vi "CreatePostUUTSequence.vi"(0 "Engine In":refnum<k7>, 5 "NewSequenceFile in":refnum<k7>, 11 "Error In":errorcluster) -> (4 "Engine Out":refnum<k7>, 6 "NewSequenceFile out":refnum<k7>, 15 "Error Out":errorcluster)   [LabVIEW 2021, in "Create Sequence.lvlib"]
uses:
  Create Sequence.lvlib
  TypeDef/StepProperties.ctl
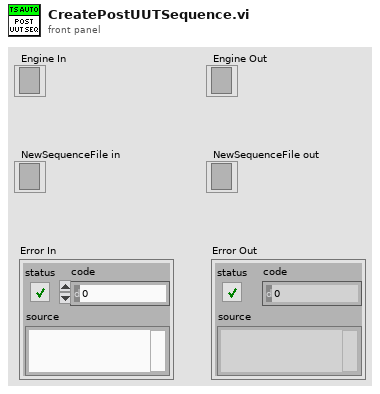
[diagram p1: front panel]
types:
  T1 = typedef "Create Sequence.lvlib/StepProperties.ctl" = cluster{"StepTypeName":string, "StepName":string, "Description":string, "Comment":string, "sequenceNameParam":string, "Step Group":i32, "Step Index":i32, "Expression":string}
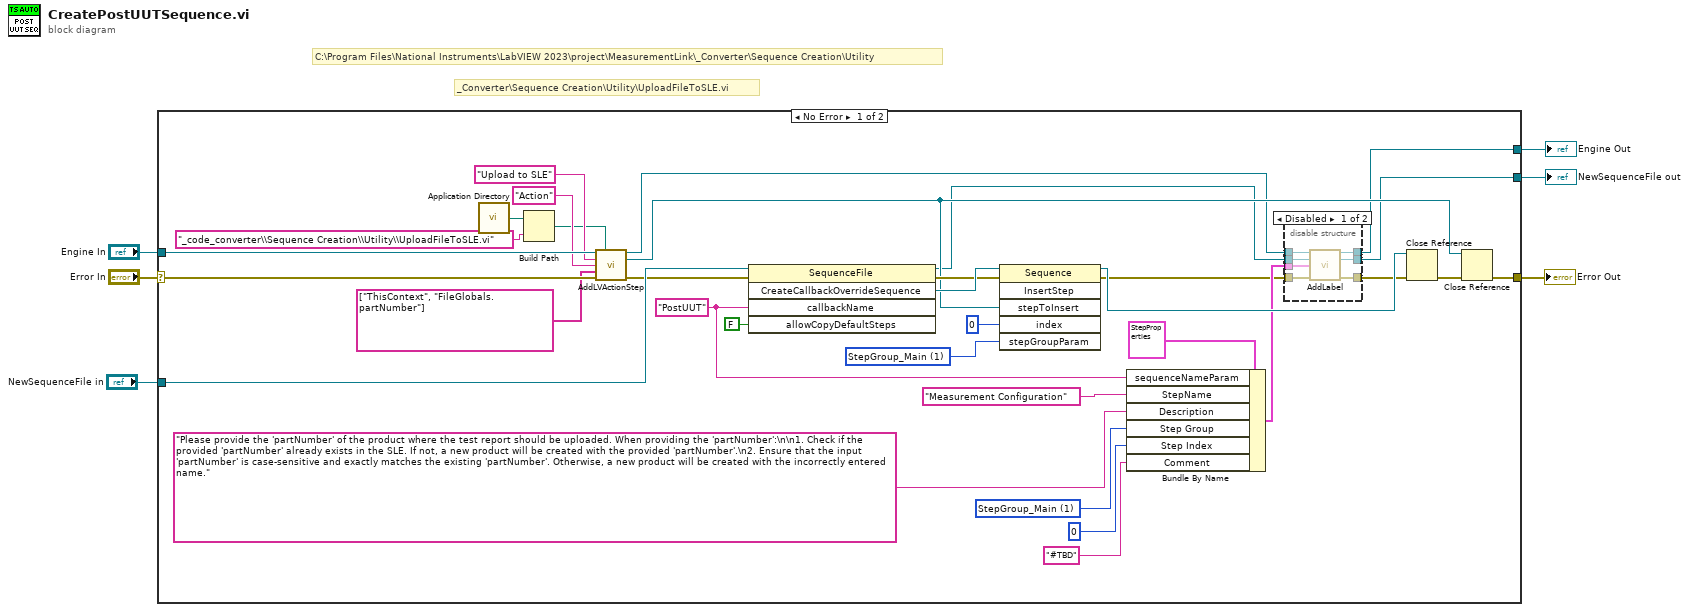
[diagram p0: block diagram]
diagram:
  # "_Converter\\Sequence Creation\\Utility\\UploadFileToSLE.vi"
  # "C:\\Program Files\\National Instruments\\LabVIEW 2023\\project\\MeasurementLink\\_Converter\\Sequence Creation\\Utility"
  n1 = case shown="No Error" "Error In" {
    selector: "Error In" -> [w35 w52]
    tunnel: [w37 w52] -> w6
    tunnel: [w11 w50] -> w5
    tunnel: [w13 w51] -> w4
    tunnel: "NewSequenceFile in" -> [w25 w50]
    tunnel: "Engine In" -> [w36 w51]
    frame No Error {
      w19 = 1 items=["StepGroup_Setup", "StepGroup_Main", "StepGroup_Cleanup"] ("Step Group")
      w28 = 1 items=["StepGroup_Setup", "StepGroup_Main", "StepGroup_Cleanup"] ("Step Group")
      w10 = "PostUUT" ("sequenceNameParam")
      n2 = call <vilib>:"Application Directory.vi"() -> ("Application Directory"=w9:path)
      n3 = Build Path(base path=w9, name or relative path="_code_converter\\Sequence Creation\\Utility\\UploadFileToSLE.vi" ("Step Type Name")) -> (appended path=w8:path)
      n4 = call "AddLVActionStep.vi"("Engine In"=w36, "VI Path"=w8, "Step Name"="Upload to SLE" ("Step Type Name"), "Step Type Name"="Action", "Parameter Value Expression"=string[] ["ThisContext", "FileGlobals.partNumber"] ("sequenceNameParam"), "Error In"=w35) -> ("Engine Out"=w14:refnum<k7>, "Step"=w31:refnum<k7>, "Error Out"=w24:errorcluster)  [unwired: 7 in]
      n5 = invoke class="SequenceFile" method="CreateCallbackOverrideSequence"(reference=w25, error in=w24, "callbackName"=w10, "allowCopyDefaultSteps"=FALSE) -> (reference out=w12:refnum<k7>, error out=w32:errorcluster, "CreateCallbackOverrideSequence"=w34:refnum<k7>)  [unwired: 1 in, 2 out]
      n6 = invoke class="Sequence" method="InsertStep"(reference=w34, error in=w32, "stepToInsert"=w31, "index"=0 ("Step Index"), "stepGroupParam"=w28) -> (reference out=w38:refnum<k7>, error out=w16:errorcluster)  [unwired: 1 in, 4 out]
      n7 = Bundle By Name(cluster=T1 {"StepTypeName"="", "StepName"="", "Description"="", "Comment"="", "sequenceNameParam"="MainSequence", "Step Group"=0, "Step Index"=3, "Expression"=""} ("StepProperties"), "sequenceNameParam"=w10, "StepName"="Measurement Configuration" ("Step Name"), "Description"="Please provide the 'partNumber' of the product where the test report should be uploaded. When providing the 'partNumber':\n\n1. Check if the provided 'partNumber' already exists in the SLE. If not, a new product will be created with the provided 'partNumber'.\n2. Ensure that the input 'partNumber' is case-sensitive and exactly matches the existing 'partNumber'. Otherwise, a new product will be created with the incorrectly entered name.", "Step Group"=w19, "Step Index"=0, "Comment"="#TBD") -> (w23:T1)
      n8 = disable-structure shown="Disabled" {
        disable-tunnel: w23 -> [w46 _]
        disable-tunnel: w16 -> [w45 w47]
        disable-tunnel: [w44 w47] -> w15
        disable-tunnel: w14 -> [w43 w49]
        disable-tunnel: [w42 w49] -> w13
        disable-tunnel: w12 -> [w41 w48]
        disable-tunnel: [w40 w48] -> w11
        frame Disabled {
          n9 = call "AddLabel.vi"("Engine In"=w43, "SequenceFile In"=w41, "StepProperties"=w46, "Error In"=w45) -> ("Engine Out"=w42:refnum<k7>, "SequenceFile Out"=w40:refnum<k7>, "Error Out"=w44:errorcluster)  [unwired: 9 in]
        }
        frame Enabled {
        }
      }
      n10 = Close Reference(reference=w38, error in (no error)=w15) -> (error out=w39:errorcluster)
      n11 = Close Reference(reference=w31, error in (no error)=w39) -> (error out=w37:errorcluster)
    }
    frame Error {
    }
  }
  "Error Out" <- w6
  "NewSequenceFile out" <- w5
  "Engine Out" <- w4
